vi "zv212cu1.vi"() -> ()   [LabVIEW 2019]
uses:
  <vilib>/Platform/TimedLoop/XDataNode/timing_clust.ctl
  <vilib>/Platform/TimedLoop/XDataNode/nitl_modes.ctl
  <vilib>/Platform/TimedLoop/XDataNode/wakeup.ctl
  <vilib>/platform/TimedLoop/XDataNode/XDataNode.xnode
  <vilib>/Platform/TimedLoop/XDataNode/XDNodeRunTimeDep.lvlib
panel:
  out "Numeric":dbl
  out "tb":dbl
  out "v_1":dbl
  out "e_v":dbl
  out "time":dbl
  out "Map":cluster{"Y":dbl[], "Y":dbl[]}[](graph)
  out "Start":i16
  out "v_sp":dbl
  in  "tf":dbl
  out "y":dbl
  out "x":dbl
  out "e_theta":dbl
  in  "Toa do":dbl[][](array[numeric])
  out "a":dbl
  out "duty3":dbl
  out "duty2":dbl
  out "duty1":dbl
  in  "Reset":bool
  out "V3_sp":dbl
  out "V3_ph":dbl
  out "Waveform Chart":T1(graph)
  in  "Ki":dbl
  in  "Kp":dbl
  out "V2_ph":dbl
  out "V1_ph":dbl
  out "V2_sp":dbl
  out "V1_sp":dbl
  in  "Start":bool
  out "v_fb":dbl
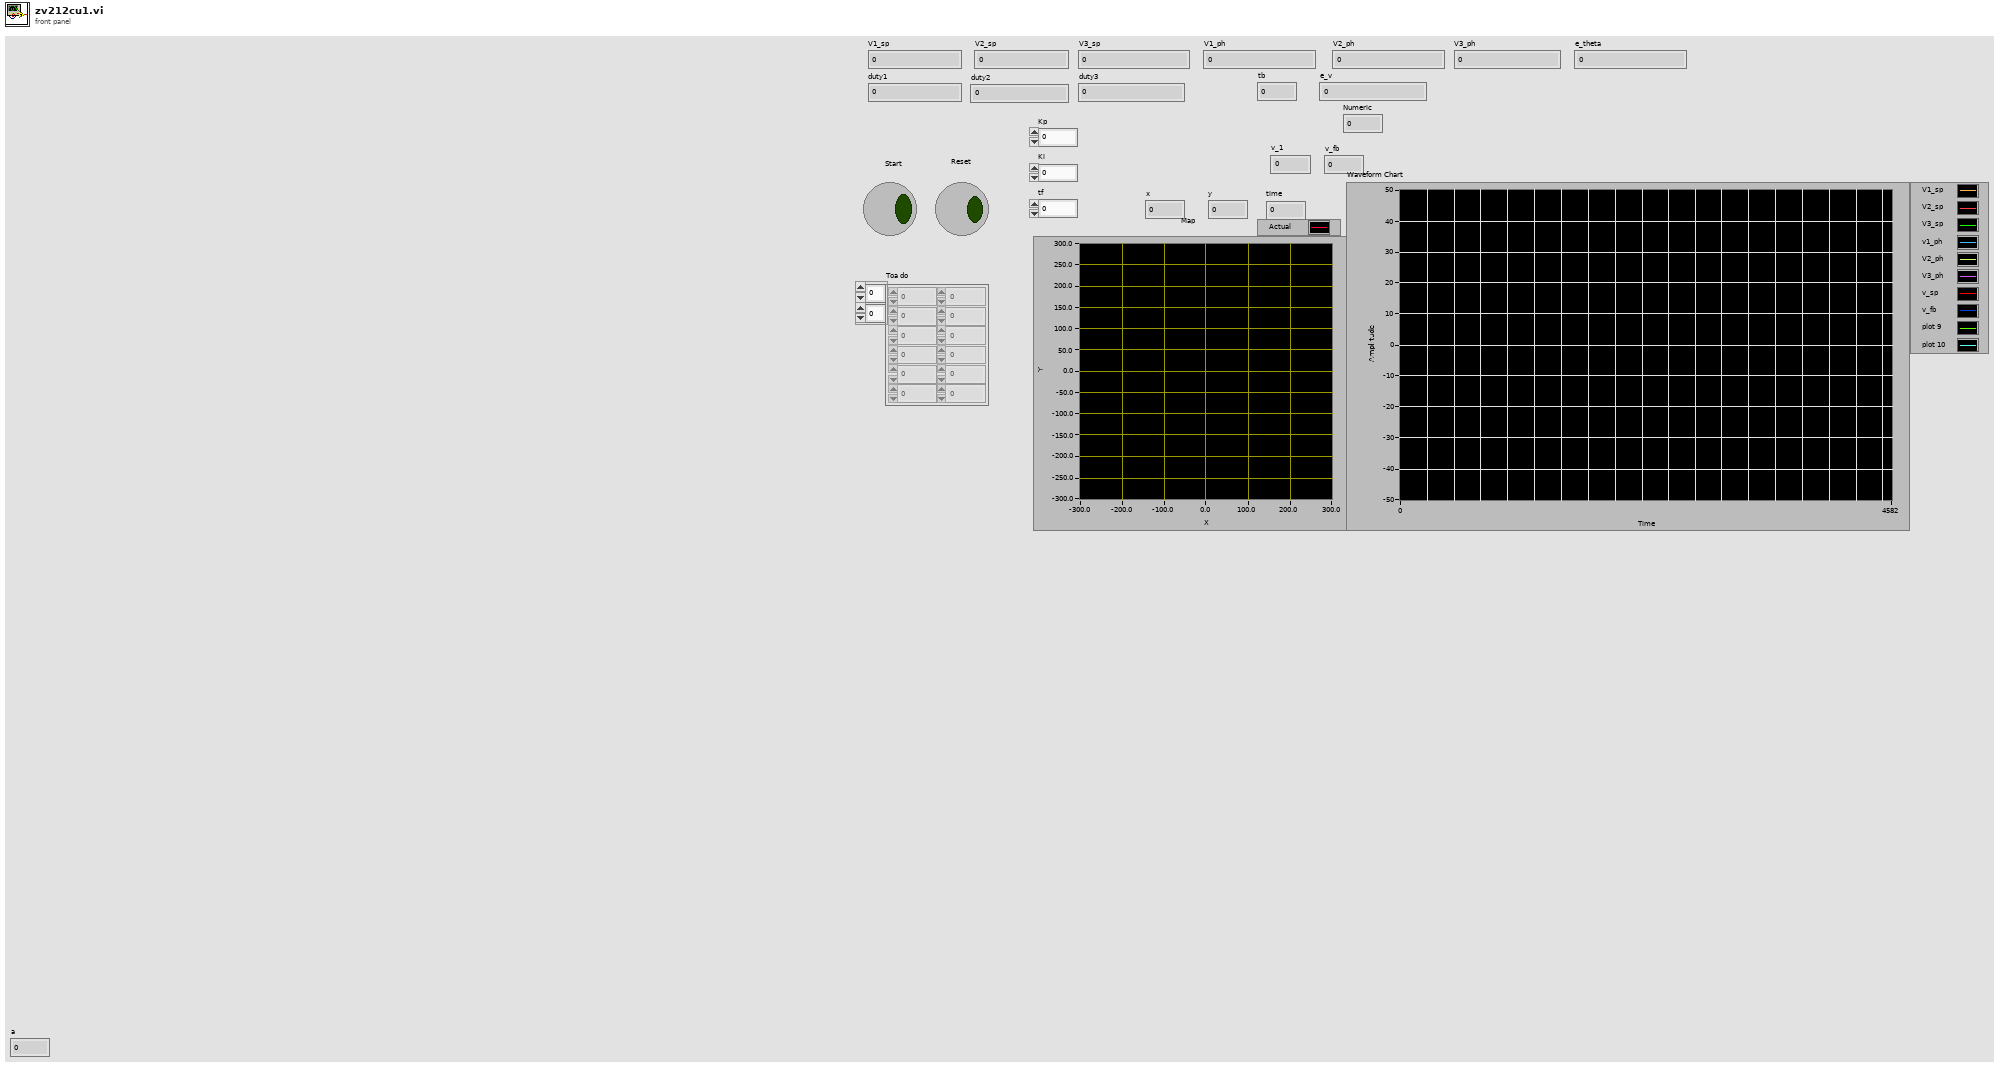
[diagram p1: front panel]
types:
  T1 = cluster{dbl, dbl, dbl, "V_ph1":dbl, "V_ph2":dbl, "V_ph3":dbl, "v_sp\n":dbl, "v_fb":dbl, dbl, "a":dbl}
  T2 = typedef "XDNodeRunTimeDep.lvlib/timing_clust.ctl" = cluster{"Expected End [f-1]":u64, "Actual End [f-1]":u64, "Finished Late? [f-1]":bool, "Expected End [i-1]":u64, "Actual End [i-1]":u64, "Finished Late? [i-1]":bool, "Expected Start [i]":u64, "Actual Start [i]":u64, "Expected Start [f]":u64, "Actual Start [f]":u64, "Source Name":string, "Structure Name":string, "Period":i64, "Deadline":i64, "Offset":i64, "Start":i64, "Priority":i32, "Timeout":i32, "Mode":T3, "Wakeup Reason":T4, "Error":errorcluster, "Source Type":string, "Secondary Source Type":string, "Global End Time":u64, "Global Start Time":u64, "Frame Duration":u64, "Iteration Duration":u64, "Assigned CPU":i32, "I/O Scan Engine Mode":u32}
  T3 = typedef "XDNodeRunTimeDep.lvlib/nitl_modes.ctl" = enum32{"No Change", "Process missed periods, maintain original phase", "Discard missed periods, maintain original phase", "Process missed periods, ignore original phase", "Discard missed periods, ignore original phase"}
  T4 = typedef "XDNodeRunTimeDep.lvlib/wakeup.ctl" = enum32{"Normal", "Aborted", "Asynchronous wakeup", "Timing source error", "Timed loop error", "Timeout"}
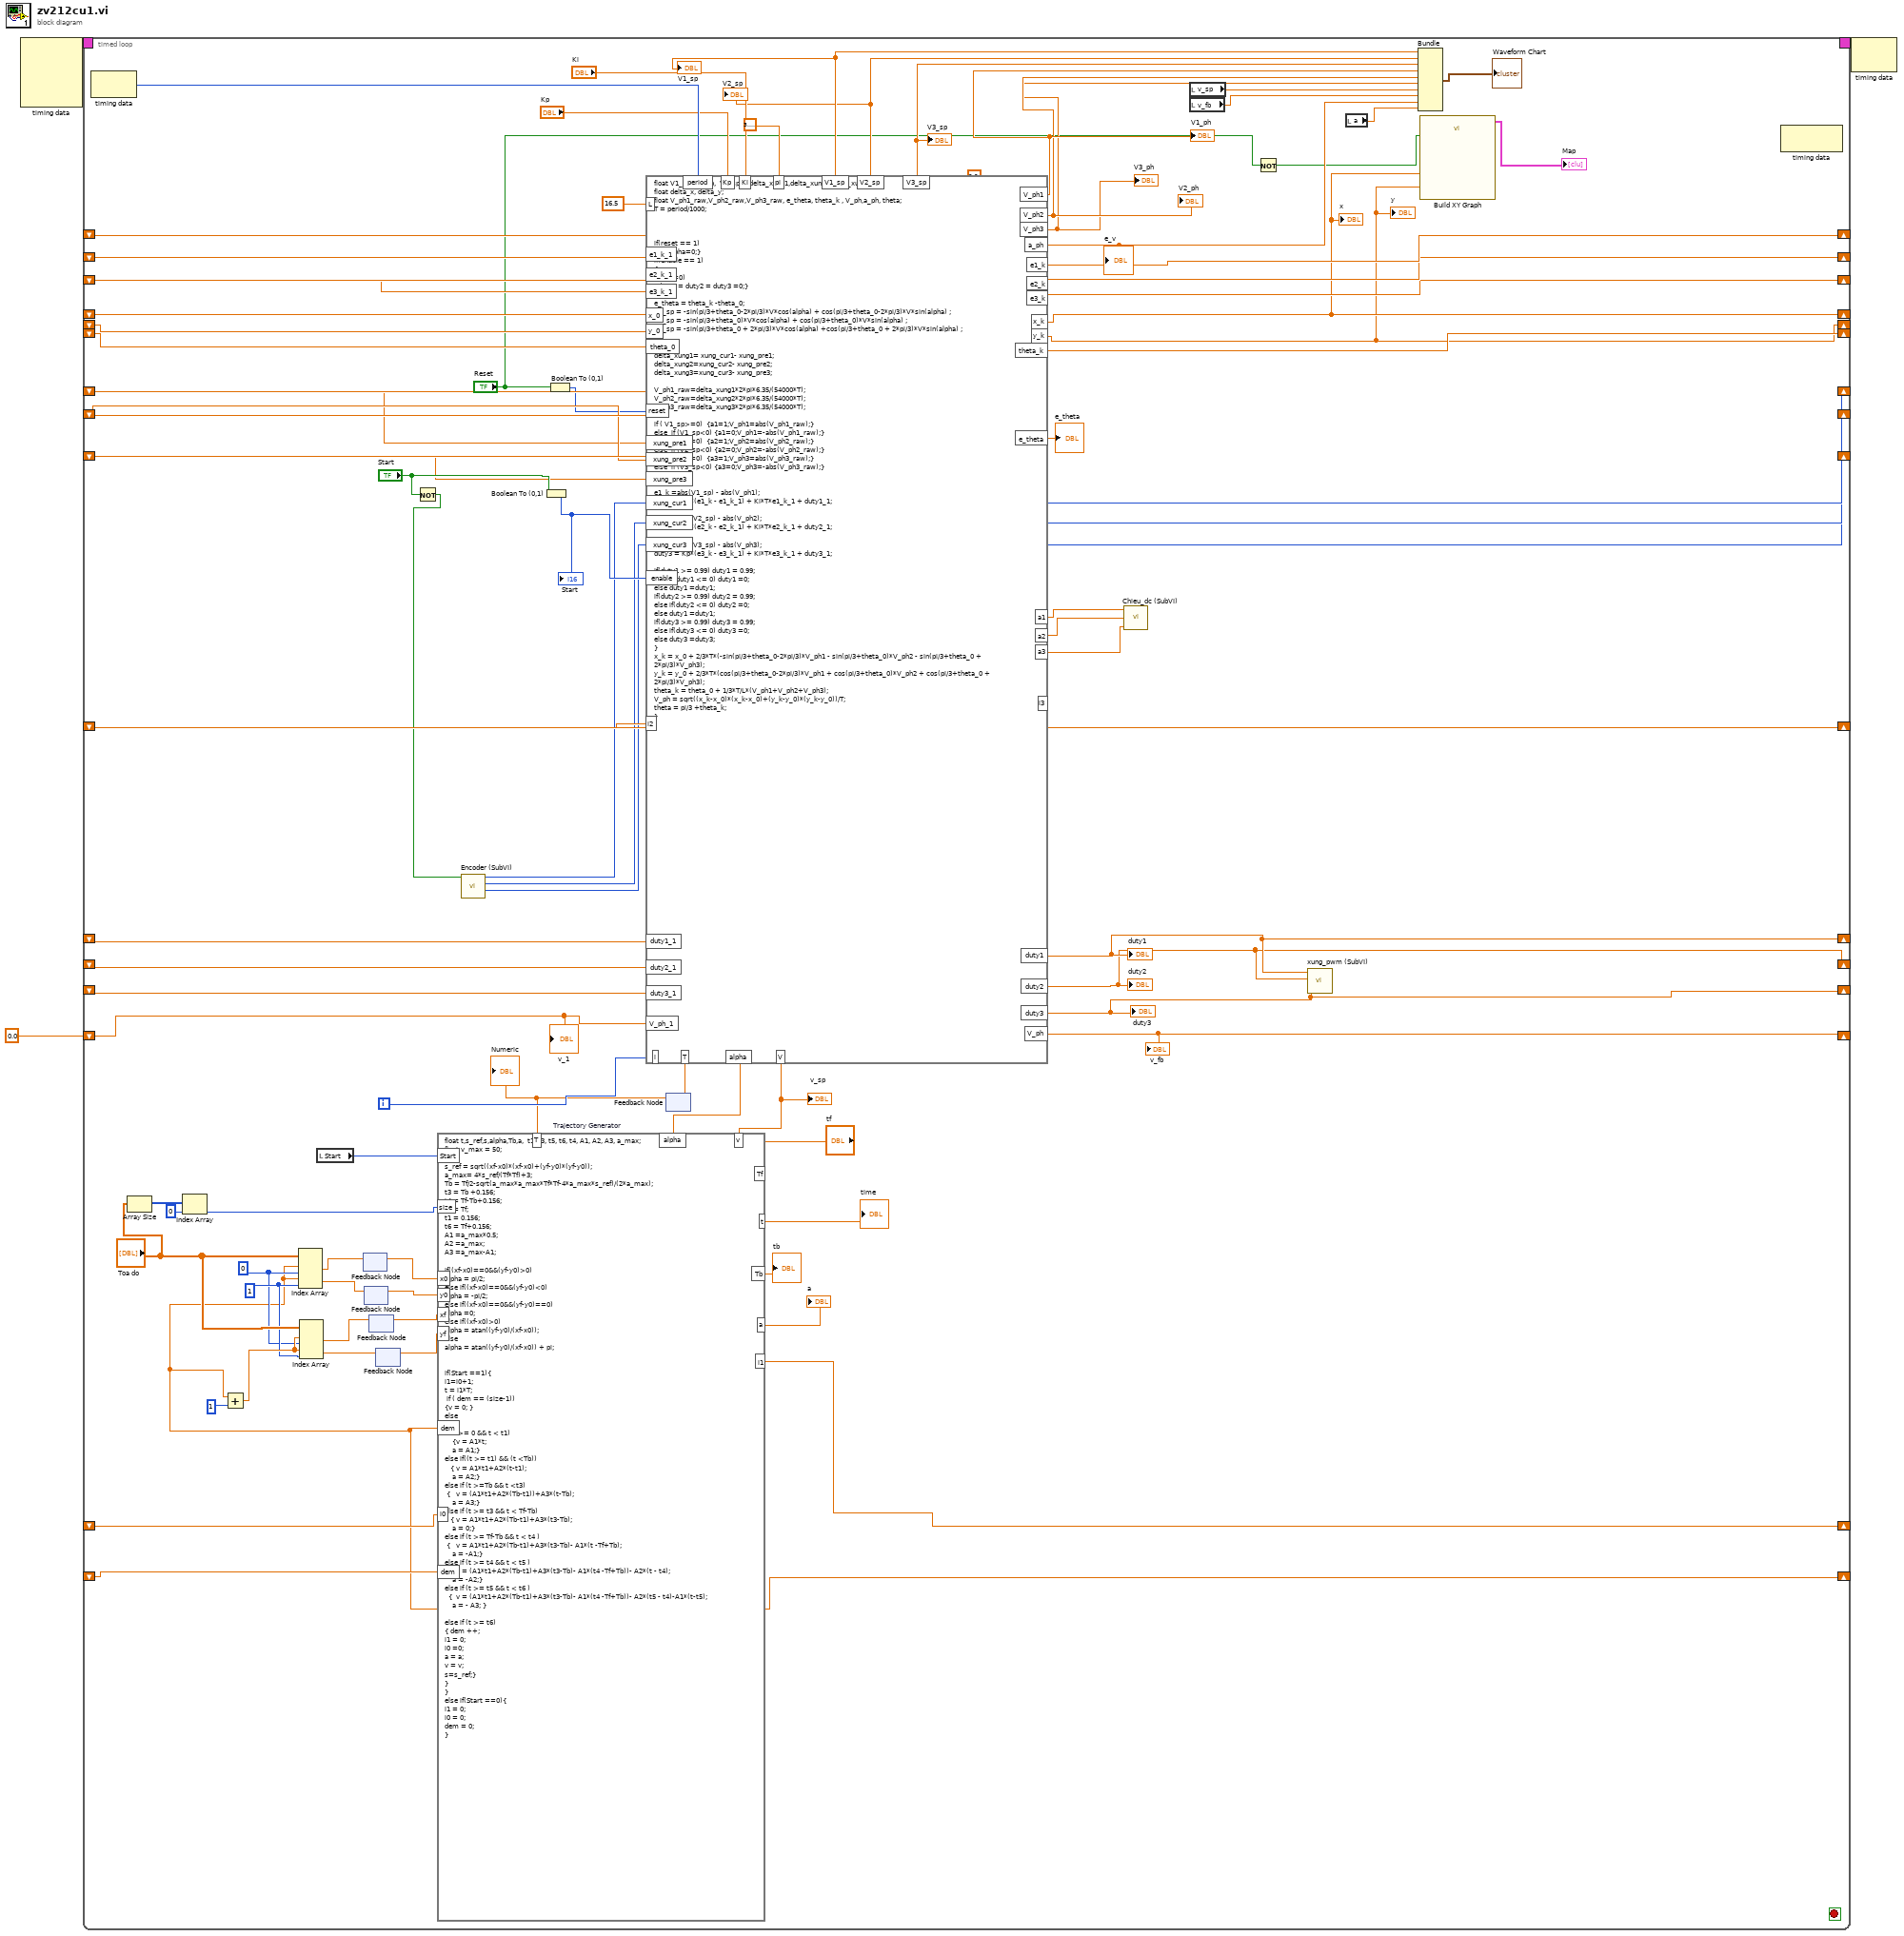
[diagram p0: block diagram]
diagram:
  w3 = 0.0 ("e1")
  n1 = node-c288() -> (w5:T2)  [unwired: 4 in]
  n2 = timed-loop {
    timing: w5 -> [_]
    timing-out: [_] -> w4
    shift-right: [w90] -> _
    shift-left: w3 -> [w88]
    shift-right: [w89] -> _
    shift-left: w3 -> [w87]
    shift-right: [w39] -> _
    shift-left: w3 -> [w76]
    shift-right: [w38] -> _
    shift-left: w3 -> [w84]
    shift-right: [w79] -> _
    shift-left: w3 -> [w78]
    shift-right: [w37] -> _
    shift-left: w3 -> [w77]
    shift-right: [w70] -> _
    shift-left: 0.0 ("i3") -> [w71]
    shift-right: [w8] -> _
    shift-left: _ -> [w69]
    shift-right: [w7] -> _
    shift-left: _ -> [w68]
    shift-right: [w6] -> _
    shift-left: _ -> [w67]
    shift-right: [w47] -> _
    shift-left: _ -> [w46]
    shift-right: [w44] -> _
    shift-left: _ -> [w45]
    shift-right: [w30] -> _
    shift-left: _ -> [w36]
    shift-right: [w29] -> _
    shift-left: _ -> [w35]
    shift-right: [w33] -> _
    shift-left: _ -> [w34]
    shift-right: [w25] -> _
    shift-left: 0.0 -> [w24]
    i -> [w66]
    stop <- _ stop-if-true
    w49 = 1
    w48 = 0
    n3 = node-c288() -> (w83:i64)  [unwired: 1 in]
    n4 = Array Size(array="Toa do") -> (size(s)=w53:i32[])
    n5 = Index Array(array=w53, index=0) -> (element=w51:i32)
    n6 = local read "Start"() -> (w16:i16)
    n7 = feedback #1() -> (w60:dbl)  [unwired: 1 in]
    n8 = feedback #2() -> (w58:dbl)  [unwired: 1 in]
    n9 = feedback #3() -> (w56:dbl)  [unwired: 1 in]
    n10 = feedback #4() -> (w54:dbl)  [unwired: 1 in]
    n11 = Not(x="Start") -> (.not. x?=w72:bool)
    n12 = call "Encoder (SubVI).vi"("Boolean"=w72) -> ("Counter Value3"=w37:i32, "Counter Value 2"=w38:i32, "Counter Value"=w39:i32)  [unwired: 8 in]
    n13 = Boolean To (0,1)(Boolean="Start") -> (0, 1=w86:i16)
    "Start" <- w86
    n14 = Boolean To (0,1)(Boolean="Reset") -> (0, 1=w74:i16)
    n15 = feedback #5() -> (w41:dbl)  [unwired: 1 in]
    "Numeric" <- w41
    n16 = formula code="float t,s_ref,s,alpha,Tb,a,  t1, t3, t5, t6, t4, A1, A2, A3, a_max;\nfloat v_max = 50;\n\ns_ref = sqrt((xf-x0)*(xf-x0)+(yf-y0)*(yf-y0));\na_max= 4*s_ref/(Tf*Tf)+3;\nTb = Tf/2-sqrt(a_max*a_max*Tf*Tf-4*a_max*s_ref)/(2*a_max);\nt3 = Tb +0.156;\nt4 = Tf-Tb+0.156;\nt5 = Tf;\nt1 = 0.156;\nt6 = Tf+0.156;\nA1 =a_max*0.5; \nA2 =a_max; \nA3 =a_max-A1;\n\nif((xf-x0)==0&&(yf-y0)>0)\nalpha = pi/2;\nelse if((xf-x0)==0&&(yf-y0)<0)\nalpha = -pi/2;\nelse if((xf-x0)==0&&(yf-y0)==0)\nalpha =0;\nelse if((xf-x0)>0)\nalpha = atan((yf-y0)/(xf-x0));\nelse \nalpha = atan((yf-y0)/(xf-x0)) + pi;\n\n\nif(Start ==1){\ni1=i0+1;\nt = i1*T;\n if ( dem == (size-1))\n{v = 0; } \nelse\n{\nif (t >= 0 && t < t1)\n    {v = A1*t;\n    a = A1;}\nelse if((t >= t1) && (t <Tb))\n   { v = A1*t1+A2*(t-t1);\n    a = A2;}\nelse if (t >=Tb && t <t3)\n {   v = (A1*t1+A2*(Tb-t1))+A3*(t-Tb);\n    a = A3;}\nelse if (t >= t3 && t < Tf-Tb)\n   { v = A1*t1+A2*(Tb-t1)+A3*(t3-Tb);\n    a = 0;}\nelse if (t >= Tf-Tb && t < t4 )\n {   v = A1*t1+A2*(Tb-t1)+A3*(t3-Tb)- A1*(t -Tf+Tb);\n    a = -A1;}\nelse if (t >= t4 && t < t5 )\n    {v = (A1*t1+A2*(Tb-t1)+A3*(t3-Tb)- A1*(t4 -Tf+Tb))- A2*(t - t4);\n    a = -A2;}\nelse if (t >= t5 && t < t6 )\n  {  v = (A1*t1+A2*(Tb-t1)+A3*(t3-Tb)- A1*(t4 -Tf+Tb))- A2*(t5 - t4)-A1*(t-t5);\n    a = - A3; }\n\nelse if (t >= t6) \n{ dem ++;\ni1 = 0;\ni0 =0;\na = a;\nv = v;\ns=s_ref;}\n}\n}\nelse if(Start ==0){\ni1 = 0;\ni0 = 0;\ndem = 0; \n}" "Trajectory Generator"("T"=w41, "Start"=w16, "Tf"="tf", "xf"=w56, "x0"=w60, "y0"=w58, "i0"=w46, "yf"=w54, "dem"=w45, "size"=w51) -> ("v"=w43:dbl, "a"=→"a":dbl, "i1"=w47:dbl, "t"=→"time":dbl, "dem"=w44:dbl, "alpha"=w40:dbl, "Tb"=→"tb":dbl)
    "v_sp" <- w43
    n17 = Add(x=w44, y=1) -> (x+y=w63:dbl)
    n18 = Index Array(array="Toa do", index (row) #1=w44, index (col) #1=w48, index (row) #2=w44, index (col) #2=w49) -> (element #1=w61:dbl, element #2=w59:dbl)
    n19 = Index Array(array="Toa do", index (row) #1=w63, index (col) #1=w48, index (row) #2=w63, index (col) #2=w49) -> (element #1=w57:dbl, element #2=w55:dbl)
    n20 = feedback-in #1(w61) -> ()
    n21 = feedback-in #2(w59) -> ()
    n22 = feedback-in #3(w57) -> ()
    n23 = feedback-in #4(w55) -> ()
    n24 = formula code="float V1_sp, V2_sp,  V3_sp,T, delta_xung1,delta_xung2,delta_xung3,S;\nfloat delta_x, delta_y;\nfloat V_ph1_raw,V_ph2_raw,V_ph3_raw, e_theta, theta_k , V_ph,a_ph, theta;\nT = period/1000;\n\n\n\nif(reset == 1)\n{V=alpha=0;}\nif(enable == 1)\n{\nif (V==0)\n{duty1 = duty2 = duty3 =0;}\nelse {\ne_theta = theta_k -theta_0;\nV1_sp = -sin(pi/3+theta_0-2*pi/3)*V*cos(alpha) + cos(pi/3+theta_0-2*pi/3)*V*sin(alpha) ;\nV2_sp = -sin(pi/3+theta_0)*V*cos(alpha) + cos(pi/3+theta_0)*V*sin(alpha) ;\nV3_sp = -sin(pi/3+theta_0 + 2*pi/3)*V*cos(alpha) +cos(pi/3+theta_0 + 2*pi/3)*V*sin(alpha) ;\n\n\ndelta_xung1= xung_cur1- xung_pre1;\ndelta_xung2=xung_cur2- xung_pre2;\ndelta_xung3=xung_cur3- xung_pre3; \n\nV_ph1_raw=delta_xung1*2*pi*6.35/(54000*T);\nV_ph2_raw=delta_xung2*2*pi*6.35/(54000*T);\nV_ph3_raw=delta_xung3*2*pi*6.35/(54000*T);\n\nif ( V1_sp>=0)  {a1=1;V_ph1=abs(V_ph1_raw);}\nelse  if (V1_sp<0) {a1=0;V_ph1=-abs(V_ph1_raw);}\nif ( V2_sp>=0)  {a2=1;V_ph2=abs(V_ph2_raw);}\nelse  if (V2_sp<0) {a2=0;V_ph2=-abs(V_ph2_raw);}\nif (V3_sp >=0)  {a3=1;V_ph3=abs(V_ph3_raw);}\nelse  if (V3_sp<0) {a3=0;V_ph3=-abs(V_ph3_raw);}\n\n\ne1_k =abs(V1_sp) - abs(V_ph1);\nduty1 = Kp*(e1_k - e1_k_1) + Ki*T*e1_k_1 + duty1_1;\n\ne2_k = abs(V2_sp) - abs(V_ph2);\nduty2 = Kp*(e2_k - e2_k_1) + Ki*T*e2_k_1 + duty2_1;\n\ne3_k = abs(V3_sp) - abs(V_ph3);\nduty3 = Kp*(e3_k - e3_k_1) + Ki*T*e3_k_1 + duty3_1;\n\nif(duty1 >= 0.99) duty1 = 0.99;\nelse if(duty1 <= 0) duty1 =0;\nelse duty1 =duty1;\nif(duty2 >= 0.99) duty2 = 0.99;\nelse if(duty2 <= 0) duty2 =0;\nelse duty1 =duty1;\nif(duty3 >= 0.99) duty3 = 0.99;\nelse if(duty3 <= 0) duty3 =0;\nelse duty3 =duty3;\n}\nx_k = x_0 + 2/3*T*(-sin(pi/3+theta_0-2*pi/3)*V_ph1 - sin(pi/3+theta_0)*V_ph2 - sin(pi/3+theta_0 + 2*pi/3)*V_ph3);\ny_k = y_0 + 2/3*T*(cos(pi/3+theta_0-2*pi/3)*V_ph1 + cos(pi/3+theta_0)*V_ph2 + cos(pi/3+theta_0 + 2*pi/3)*V_ph3);\ntheta_k = theta_0 + 1/3*T/L*(V_ph1+V_ph2+V_ph3);\nV_ph = sqrt((x_k-x_0)*(x_k-x_0)+(y_k-y_0)*(y_k-y_0))/T;\ntheta = pi/3 +theta_k;\n}"("Kp"="Kp", "Ki"="Ki", "pi"=3.141592653589793, "e1_k_1"=w88, "e2_k_1"=w87, "xung_pre1"=w76, "xung_pre2"=w84, "xung_cur1"=w39, "xung_cur2"=w38, "enable"=w86, "period"=w83, "e3_k_1"=w78, "xung_cur3"=w37, "xung_pre3"=w77, "reset"=w74, "i"=w66, "i2"=w71, "duty1_1"=w69, "duty2_1"=w68, "duty3_1"=w67, "alpha"=w40, "V"=w43, "x_0"=w36, "y_0"=w35, "theta_0"=w34, "L"=16.5, "V_ph_1"=w24) -> ("V1_sp"=w73:dbl, "V_ph1"=w20:dbl, "V_ph2"=w19:dbl, "e1_k"=w90:dbl, "e2_k"=w89:dbl, "V2_sp"=w22:dbl, "duty1"=w8:dbl, "duty2"=w7:dbl, "e3_k"=w79:dbl, "V_ph3"=w18:dbl, "V3_sp"=w21:dbl, "duty3"=w6:dbl, "a1"=w28:dbl, "a2"=w27:dbl, "a3"=w26:dbl, "i3"=w70:dbl, "T"=w42:dbl, "x_k"=w30:dbl, "y_k"=w29:dbl, "theta_k"=w33:dbl, "e_theta"=→"e_theta":dbl, "V_ph"=w25:dbl, "a_ph"=w14:dbl)
    "V1_sp" <- w73
    "V2_sp" <- w22
    "V1_ph" <- w20
    "V2_ph" <- w19
    "V3_ph" <- w18
    "V3_sp" <- w21
    "duty1" <- w8
    "duty2" <- w7
    "duty3" <- w6
    "x" <- w30
    "y" <- w29
    "v_fb" <- w25
    "e_v" <- w14
    n25 = feedback-in #5(w42) -> ()
    n26 = call "Chieu_dc (SubVI).vi"("a3"=w26, "a2"=w27, "a1"=w28) -> ()
    n27 = local read "v_sp"() -> (w17:dbl)
    n28 = local read "v_fb"() -> (w15:dbl)
    n29 = Not(x="Reset") -> (.not. x?=w10:bool)
    n30 = call "xung_pwm (SubVI).vi"("duty3 in"=w6, "duty2 in"=w7, "duty1 in"=w8) -> ()  [unwired: 6 in, 3 out]
    n31 = local read "a"() -> (w13:dbl)
    n32 = Bundle(w73, w22, w21, "V_ph1"=w20, "V_ph2"=w19, "V_ph3"=w18, "v_sp"=w17, "v_fb"=w15, w14, "a"=w13) -> (→"Waveform Chart":T1)  [unwired: 1 in]
    n33 = call "Build XY Graph"("Reset"=w10, "Y Input"=w29, "X Input"=w30) -> ("XY Graph"=→"Map":cluster{"X":dbl[], "Y":dbl[]}[])  [unwired: 7 in, 1 out]
    n34 = node-c288() -> ()  [unwired: 1 in, 1 out]
    "v_1" <- w24
  }
  n35 = node-c288(w4) -> ()  [unwired: 1 out]
